vi "UsrProfiles-Check profile belongs to selected user.vi"(11 "Filename of loaded user profile":string) -> (1 "Belongs to selected user":bool)   [LabVIEW 2017]
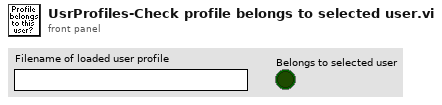
[diagram p1: front panel]
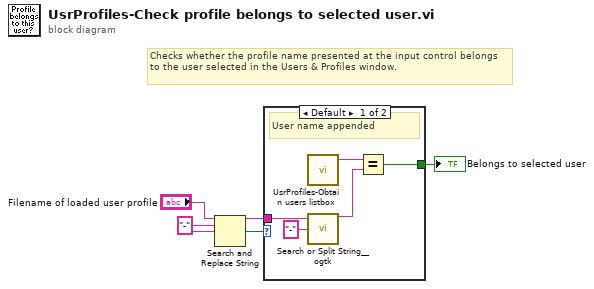
[diagram p0: block diagram]
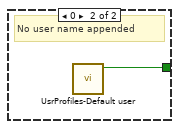
[diagram p2: hidden frame]
diagram:
  w5 = "-" ("search string")
  # "Checks whether the profile name presented at the input control belongs to the user selected in the Users & Profiles window."
  n1 = Search and Replace String(input string="Filename of loaded user profile", search string=w5, replace string=w5) -> (result string=w3:string, number of replacements=w4:i32)  [unwired: 5 in, 2 out]
  n2 = case shown="Default" w4 {
    tunnel: w3 -> [w9 _]
    tunnel: [w7 w11] -> w1
    frame Default {
      # "User name appended"
      n3 = call "UsrProfiles-Obtain users listbox.vi"() -> ("Selected user's name"=w6:string)  [unwired: 8 in, 3 out]
      n4 = call <userlib>:"Search or Split String__ogtk.vi"("search string/char (-)"="-", "string"=w9) -> ("substring before match"=w8:string)  [unwired: 1 in, 2 out]
      n5 = Equal?(x=w6, y=w8) -> (x = y?=w7:bool)
    }
    frame 0 {
      # "No user name appended"
      n6 = call "UsrProfiles-Default user.vi"() -> ("Default user selected"=w11:bool)  [unwired: 9 in, 2 out]
    }
  }
  "Belongs to selected user" <- w1
